vi "I2C An Out 0-20mA(GP8313).vi"() -> ()   [LabVIEW 2020, in "CTI-Scratchpad.lvlib"]
uses:
  CTI-Scratchpad.lvlib
  CTI/Identity.ctl
  CTI/Error Reporting.ctl
  CTI/GPIO Number.ctl
  CTI/I2C Number.ctl
  CTI/Session/Session.lvclass
  CTI-Peripheral/Analog Output/1 Chan I2C An Out/I2C_0-20mA(GP8313)/I2C_0-20mA(GP8313).lvclass
  CTI/VisaComms/VisaComms.lvclass
  CTI/CTI.lvlib
panel:
  in  "V0":u16(slide)=2000 scale=0.0..32767.0
  out "loop":i32
  in  "stop":bool
  out "Identity":T1
  in  "Grove Connector":enum16{"I2C0", "I2C1"}(ring)
  out "error out":errorcluster
  in  "Port":refnum<visa-resource-name>="COM4"
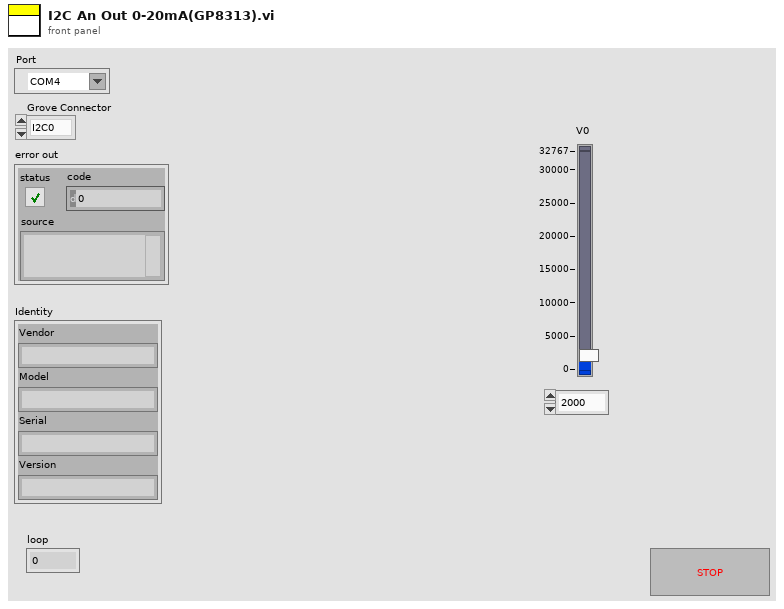
[diagram p1: front panel]
types:
  T1 = typedef "CTI.lvlib/Identity.ctl" = cluster{"Vendor":string, "Model":string, "Serial":string, "Version":string}
  T2 = typedef "CTI.lvlib/Error Reporting.ctl" = enum16{"Minimal", "Moderate", "Full"}
  T3 = typedef "CTI.lvlib/I2C Number.ctl" = i8
  T4 = typedef "CTI.lvlib/GPIO Number.ctl" = i8
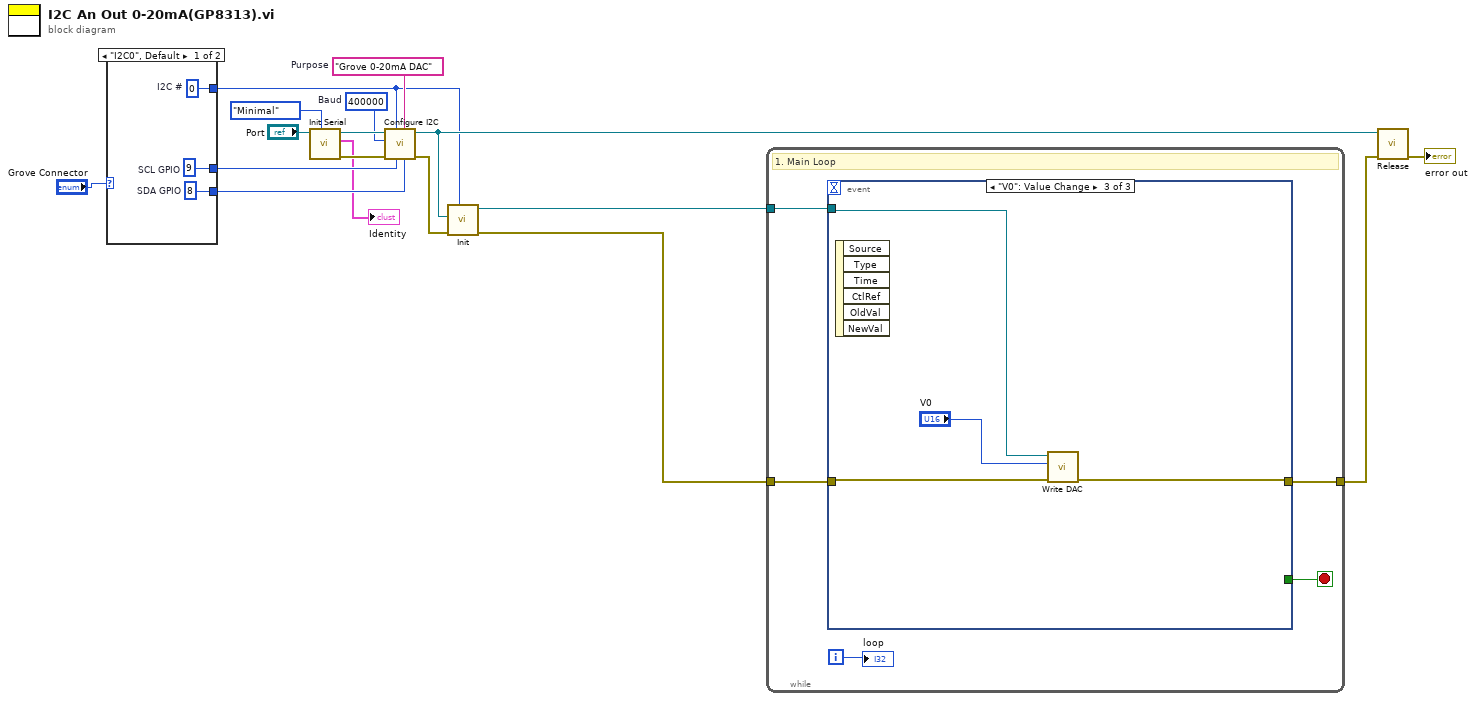
[diagram p0: block diagram]
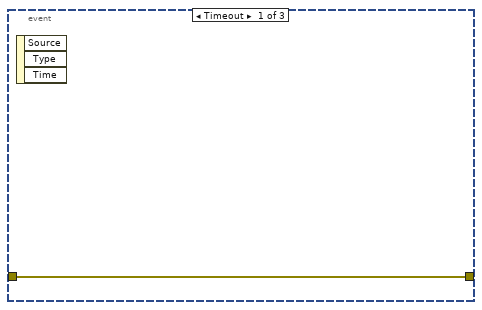
[diagram p2: hidden frame]
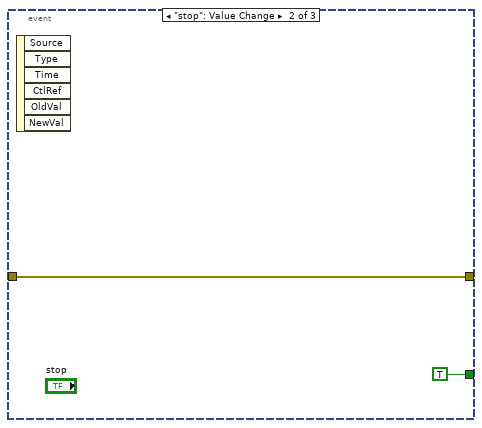
[diagram p3: hidden frame]
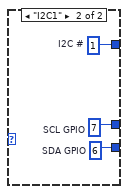
[diagram p4: hidden frame]
diagram:
  w12 = "Grove 0-20mA DAC"  # Purpose
  w13 = u32 400000  # Baud
  n1 = case shown="\"I2C0\", Default" "Grove Connector" {
    tunnel: [w20 w23] -> w10
    tunnel: [w19 w22] -> w9
    tunnel: [w18 w21] -> w3
    frame "I2C0", Default {
      w18 = T3 0  # I2C #
      w19 = T4 8  # SDA GPIO
      w20 = T4 9  # SCL GPIO
    }
    frame "I2C1" {
      w21 = T3 1  # I2C #
      w22 = T4 6  # SDA GPIO
      w23 = T4 7  # SCL GPIO
    }
  }
  n2 = call "Init Serial.vi"("Error Checking (Full)"=Error_Reporting."Minimal", "VISA resource name in"="Port") -> ("error out"=w14:errorcluster, "Identity"=→"Identity":T1, "Session"=w15:refnum<class "Session.lvclass">)  [unwired: 7 in]
  n3 = call "Configure I2C.vi"("SDA GPIO"=w9, "Purpose (\"I2C\")"=w12, "SCL GPIO"=w10, "I2C #"=w3, "error in (no error)"=w14, "Baud"=w13, "Session in"=w15) -> ("error out"=w4:errorcluster, "Session out"=w5:refnum<class "Session.lvclass">)  [unwired: 3 in]
  n4 = call "Init.vi"("I2C #"=w3, "error in (no error)"=w4, "Session In"=w5) -> ("error out"=w1:errorcluster, "I2C_0-20mA(GP8313) Out"=w2:refnum<class "I2C_0-20mA(GP8313).lvclass">)  [unwired: 7 in]
  n5 = while {
    tunnel: w1 -> [w27]
    tunnel: w2 -> [w28]
    tunnel: [w25] -> w7
    i -> [w26]
    stop <- w24 stop-if-true
    # "1. Main Loop"
    n6 = event shown="[2] \"V0\": Value Change" {
      selector: _ -> [_ _ _]
      dyn-events: _ -> [_ _ _]
      timeout: _ -> [_ _ _]
      tunnel: w28 -> [_ _ w33]
      tunnel: w27 -> [w29 w30 w35]
      tunnel: [w29 w30 w34] -> w25
      tunnel: [_ TRUE _] -> w24
      event Timeout {
        n7 = event-data() -> ()  [unwired: 1 in, 3 out]
      }
      event "stop": Value Change {
        n8 = event-data() -> ()  [unwired: 1 in, 6 out]
      }
      event "V0": Value Change {
        n9 = event-data() -> ()  [unwired: 1 in, 6 out]
        n10 = call-dynamic "Write DAC.vi"("error in (no error)"=w35, "Analog Output"="V0", "I2C_0-20mA(GP8313) in"=w33) -> ("error out"=w34:errorcluster)  [unwired: 7 in, 1 out]
      }
    }
    "loop" <- w26
  }
  n11 = call-dynamic "Release.vi"("error in (no error)"=w7, "Session in"=w5) -> ("error out"=→"error out":errorcluster)  [unwired: 9 in]
